vi "Get Channel Names from Channel Table.vi"(11 "Channel Table":T1[](array[typedef]) {"input terminal configuration" items=["default"=-1, "RSE"=10083, "NRSE"=10078, "Differential"=10106, "Pseudodifferential"=12529]; "Channel Type" items=["Voltage (V)"=0, "Charge (C)"=9, "-"=99, "SPL (Pa)"=3, "Force (lbf)"=6, "Force (N)"=1, "Acceleration (g) - IEPE"=2, "Acceleration (g) - Charge"=12, "Acceleration (g) - 4 wire DC Voltage"=22, "Velocity (in/s)"=7, "Velocity (mm/s)"=8, "Prox Probe (mil)"=4, "Prox Probe (mm)"=5]}) -> (3 "All Channels":string[](array[string]))   [LabVIEW 2024, in "Dynamic Signal Acquisition (Interactive) UI.lvlib"]
uses:
  Dynamic Signal Acquisition (Interactive) UI.lvlib
  <vilib>/addons/Sound and Vibration/svt_DAQmx/Configuration XControl/SVX NI-DAQmx AI Configuration XControl.xctl
  SFPDAQmx Channel Info.ctl
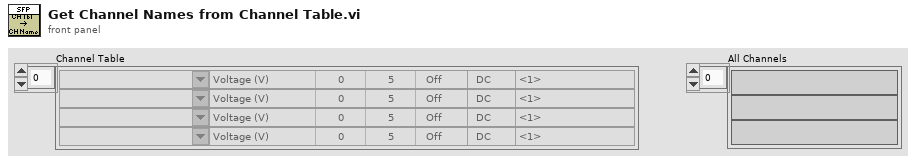
[diagram p1: front panel]
types:
  T1 = typedef "Dynamic Signal Acquisition (Interactive) UI.lvlib/SFPDAQmx Channel Info.ctl" = cluster{"Initialized?":bool, "DAQmx Channel":tag, "Channel Type":u16, "Max":dbl, "Sensitivity":dbl, "Excitation":bool, "Coupling":enum16{"AC", "DC"}, "input terminal configuration":i32, "excitation":enum16{"Off", "Min", "Max"}}
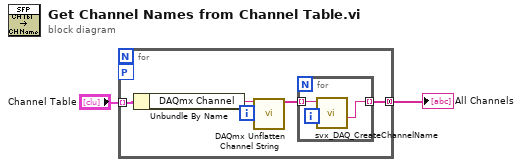
[diagram p0: block diagram]
diagram:
  n1 = for {
    tunnel: "Channel Table" -> [w6] mode=indexing
    workers-P: _ -> [_]
    tunnel: [w5] -> w1 mode=concatenating
    n2 = Unbundle By Name(w6) -> ("DAQmx Channel"=w4:tag)
    n3 = call <vilib>:"DAQmx Unflatten Channel String.vi"("names in"=w4) -> ("names out"=w3:string[])  [unwired: 13 in, 1 out]
    n4 = for {
      tunnel: [w7] -> w5 mode=indexing
      tunnel: w3 -> [w8] mode=indexing
      n5 = call <vilib>:"svx_DAQ_CreateChannelName.vi"("DAQmx Channel In"=w8) -> ("Channel Name"=w7:string)  [unwired: 9 in, 1 out]
    }
  }
  "All Channels" <- w1
